vi "LCR Meter Acquire Single_1.vi"() -> ()   [LabVIEW 2021, in "LCR Meter.lvlib"]
doc: "This example shows how to configure a measurement and take a reading."
uses:
  <vilib>/LCR Meter.lvlib
panel:
  out "Boolean":bool
  out "Monitor2 Value":dbl
  out "Monitor1 Value":dbl
  out "Secondary Value":dbl
  out "Primary Value":dbl
  in  "DC Bias Voltage (0)":dbl min=-2.5 max=2.5 step=0.01
  in  "DC Bias":bool caption="BIAS"
  in  "Current Level (1)":dbl=1.0 min=0.1 max=20.0 step=0.01
  in  "Voltage Level (1)":dbl=1.0 min=0.01 max=2.0 step=0.01
  in  "Level Mode":u16(ring) items=["Voltage", "Current"]
  in  "ALC (F: Disable)":bool
  in  "Frequery (1000)":dbl=1000.0 min=10.0 max=300000.0 step=0.01
  in  "Monitor2":i32(ring) items=["OFF", "Z", "D", "Q", "THR", "THD", "R", "X", "G", "B", "Y", "ABS", "PER", "VAC", "IAC"]
  in  "Monitor1":i32(ring) items=["OFF", "Z", "D", "Q", "THR", "THD", "R", "X", "G", "B", "Y", "ABS", "PER", "VAC", "IAC"]
  in  "Speed (0: SLOW)":i32(ring) items=["SLOW", "MED", "FAST"]
  in  "Average (0)":i32 min=0 max=256 step=1
  in  "Auto Range (1: ON)":i32(ring)=1 items=["OFF", "ON", "NOM"]
  in  "Range (0: 0)":i32(ring) items=["0", "1", "2", "3", "4", "5", "6", "7", "8", "MIN", "MAX"]
  in  "Auto LCZ (T: Enable)":bool=TRUE
  in  "Function (0: Cs-Rs)":i32(ring) items=["Cs-Rs", "Cs-D", "Cp-Rp", "Cp-D", "Lp-Rp", "Lp-Q", "Ls-Rs", "Ls-Q", "Rs-Q", "Rp-Q", "R-X", "DCR", "Z-thr", "Z-thd", "Z-D", "Z-Q"]
  in  "Serial Settings:Baud Rate":u32(ring)=115200 items=["9600"=9600, "38400"=38400, "57600"=57600, "115200"=115200]
  in  "VISA resource name":refnum<visa-resource-name>
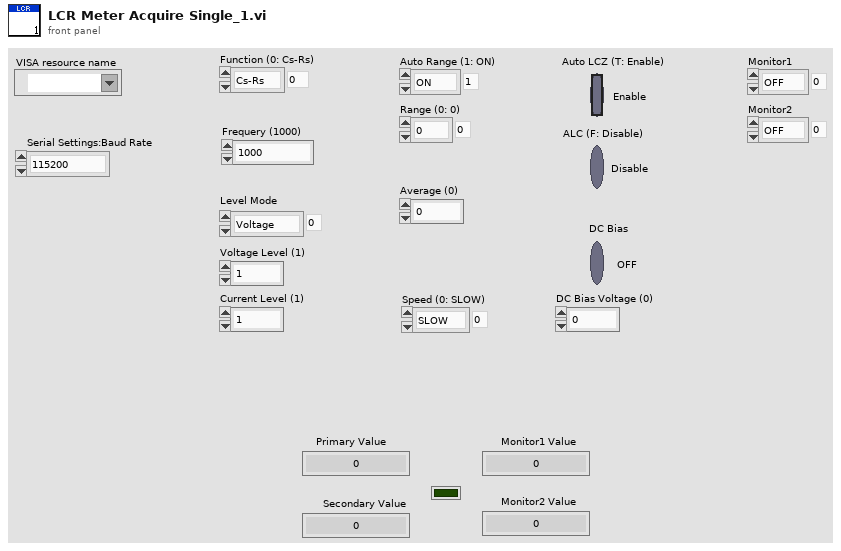
[diagram p1: front panel]
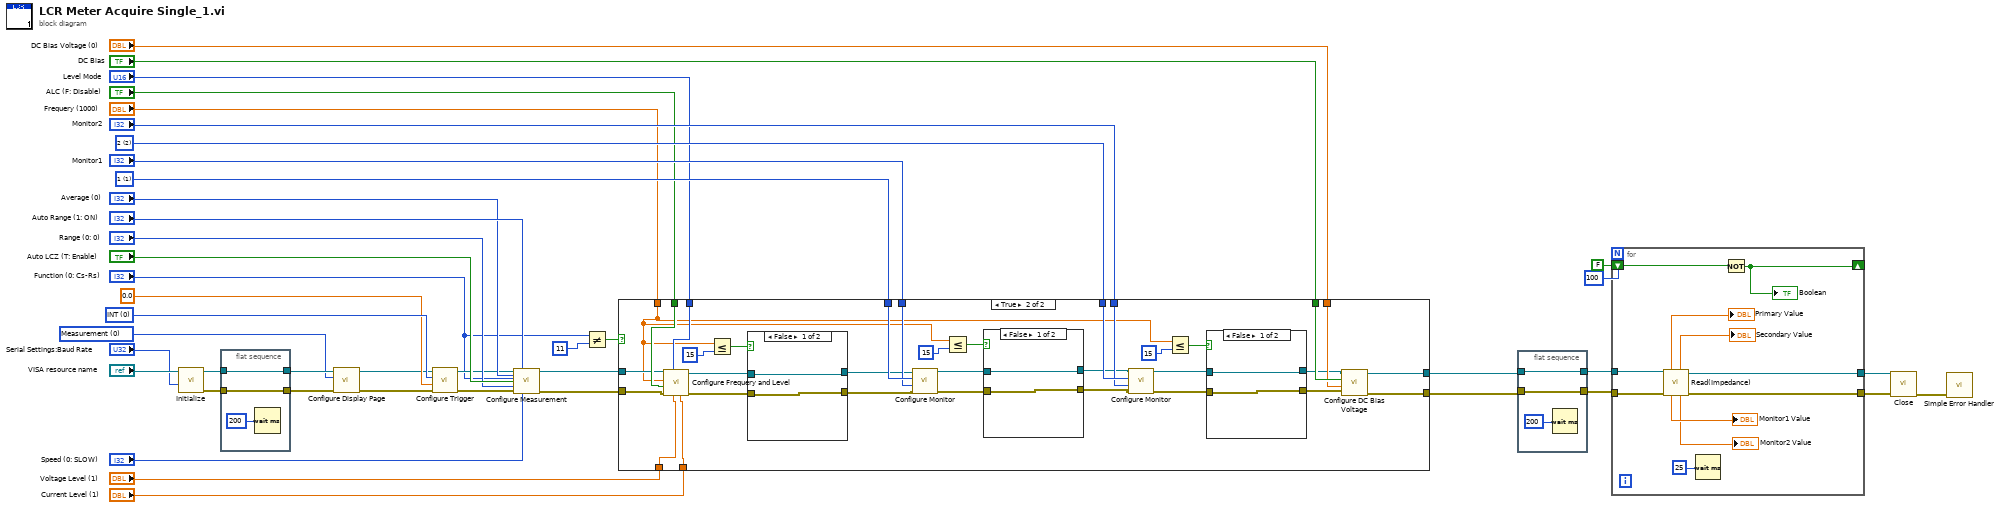
[diagram p0: block diagram]
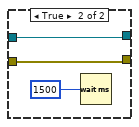
[diagram p3: hidden frame]
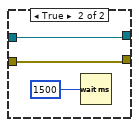
[diagram p4: hidden frame]
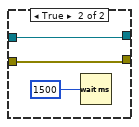
[diagram p5: hidden frame]
diagram:
  w10 = u16 0 items=["Measurement", "Measurement Setup", "BIN Measurement", "BIN Count", "BIN Setup", "LIST Measurement", "LIST Setup", "CORRECTION", "CATALOG", "ENLARGE", "System Config", "System Information"] ("Display Page")
  w22 = 0 items=["INT", "MAN", "EXT", "BUS"] ("Trigger Source (0: INT)")
  w32 = 2 items=["1"=1, "2"=2] ("Monitor (1)")
  w34 = 1 items=["1"=1, "2"=2] ("Monitor (1)")
  n1 = call <vilib>:"Initialize.vi"("Serial Settings:Baud Rate"="Serial Settings:Baud Rate", "VISA resource name"="VISA resource name") -> ("error out"=w13:errorcluster, "VISA resource name out"=w16:refnum<visa-resource-name>)  [unwired: 7 in, 1 out]
  n2 = flat-sequence {
    tunnel: [w46] -> w15
    tunnel: w16 -> [w46]
    tunnel: w13 -> [w45]
    tunnel: [w45] -> w12
    frame #0 {
      n3 = Wait (ms)(milliseconds to wait=u32 200) -> ()  [unwired: 1 out]
    }
  }
  n4 = call <vilib>:"Configure Display Page.vi"("error in"=w12, "Display Page"=w10, "VISA resource name"=w15) -> ("error out"=w11:errorcluster, "VISA resource name out"=w14:refnum<visa-resource-name>)  [unwired: 7 in]
  n5 = call <vilib>:"Configure Trigger.vi"("error in (no error)"=w11, "Trigger Delay (0)"=0.0, "Trigger Source (0: INT)"=w22, "VISA resource name"=w14) -> ("error out"=w23:errorcluster, "VISA resource name out"=w24:refnum<visa-resource-name>)  [unwired: 6 in]
  n6 = call <vilib>:"Configure Measurement.vi"("VISA resource name"=w24, "Auto Range (1: ON)"="Auto Range (1: ON)", "Average (0)"="Average (0)", "Function (0: Cs-Rs)"="Function (0: Cs-Rs)", "Auto LCZ (T: Enable)"="Auto LCZ (T: Enable)", "Range (0: 0)"="Range (0: 0)", "error in (no error)"=w23, "Speed (0: SLOW)"="Speed (0: SLOW)") -> ("VISA resource name out"=w36:refnum<visa-resource-name>, "error out"=w35:errorcluster)  [unwired: 6 in]
  n7 = Not Equal?(x="Function (0: Cs-Rs)", y=11) -> (x != y?=w9:bool)
  n8 = case shown="True" w9 {
    tunnel: w36 -> [w48 w69]
    tunnel: w35 -> [w47 w68]
    tunnel: w34 -> [_ w81]
    tunnel: "Monitor1" -> [_ w80]
    tunnel: w32 -> [_ w79]
    tunnel: "Monitor2" -> [_ w78]
    tunnel: "Frequery (1000)" -> [_ w49]
    tunnel: "ALC (F: Disable)" -> [_ w73]
    tunnel: "Level Mode" -> [_ w72]
    tunnel: "Voltage Level (1)" -> [_ w71]
    tunnel: "Current Level (1)" -> [_ w70]
    tunnel: "DC Bias" -> [_ w77]
    tunnel: "DC Bias Voltage (0)" -> [_ w76]
    tunnel: [w48 w75] -> w5
    tunnel: [w47 w74] -> w4
    frame False {
    }
    frame True {
      n9 = call <vilib>:"Configure Frequery and Level.vi"("Current Level (1)"=w70, "Voltage Level (1)"=w71, "Level Mode"=w72, "error in (no error)"=w68, "ALC (F: Disable)"=w73, "Frequery (1000)"=w49, "VISA resource name"=w69) -> ("error out"=w65:errorcluster, "VISA resource name out"=w64:refnum<visa-resource-name>)  [unwired: 3 in]
      n10 = Less Or Equal?(x=w49, y=15) -> (x <= y?=w66:bool)
      n11 = case shown="False" w66 {
        tunnel: w64 -> [w93 w95]
        tunnel: w65 -> [w92 w94]
        tunnel: [w93 w95] -> w62
        tunnel: [w92 w94] -> w63
        frame False {
        }
        frame True {
          n12 = Wait (ms)(milliseconds to wait=u32 1500) -> ()  [unwired: 1 out]
        }
      }
      n13 = call <vilib>:"Configure Monitor.vi"("error in (no error)"=w63, "Parameter (0: OFF)"=w80, "Monitor (1)"=w81, "VISA resource name"=w62) -> ("error out"=w54:errorcluster, "VISA resource name out"=w57:refnum<visa-resource-name>)  [unwired: 6 in]
      n14 = Less Or Equal?(x=w49, y=15) -> (x <= y?=w60:bool)
      n15 = case shown="False" w60 {
        tunnel: w57 -> [w88 w90]
        tunnel: w54 -> [w87 w89]
        tunnel: [w88 w90] -> w56
        tunnel: [w87 w89] -> w53
        frame False {
        }
        frame True {
          n16 = Wait (ms)(milliseconds to wait=u32 1500) -> ()  [unwired: 1 out]
        }
      }
      n17 = call <vilib>:"Configure Monitor.vi"("error in (no error)"=w53, "Parameter (0: OFF)"=w78, "Monitor (1)"=w79, "VISA resource name"=w56) -> ("error out"=w52:errorcluster, "VISA resource name out"=w55:refnum<visa-resource-name>)  [unwired: 6 in]
      n18 = Less Or Equal?(x=w49, y=15) -> (x <= y?=w58:bool)
      n19 = case shown="False" w58 {
        tunnel: w55 -> [w83 w85]
        tunnel: w52 -> [w82 w84]
        tunnel: [w83 w85] -> w51
        tunnel: [w82 w84] -> w50
        frame False {
        }
        frame True {
          n20 = Wait (ms)(milliseconds to wait=u32 1500) -> ()  [unwired: 1 out]
        }
      }
      n21 = call <vilib>:"Configure DC Bias Voltage.vi"("VISA resource name"=w51, "DC Bias"=w77, "DC Bias Voltage (0)"=w76, "error in (no error)"=w50) -> ("VISA resource name out"=w75:refnum<visa-resource-name>, "error out"=w74:errorcluster)  [unwired: 5 in]
    }
  }
  n22 = flat-sequence {
    tunnel: [w99] -> w3
    tunnel: w5 -> [w99]
    tunnel: w4 -> [w98]
    tunnel: [w98] -> w2
    frame #0 {
      n23 = Wait (ms)(milliseconds to wait=u32 200) -> ()  [unwired: 1 out]
    }
  }
  n24 = for {
    N: 100 -> [_]
    tunnel: w2 -> [w110]
    tunnel: [w104] -> w20
    tunnel: [w103] -> w19
    shift-right: [w101] -> _
    shift-left: FALSE -> [w102]
    tunnel: w3 -> [w100]
    n25 = call <vilib>:"Read(Impedance).vi"("error in (no error)"=w110, "VISA resource name"=w100) -> ("error out"=w103:errorcluster, "VISA resource name out"=w104:refnum<visa-resource-name>, "Monitor2 Value"=→"Monitor2 Value":dbl, "Secondary Value"=→"Secondary Value":dbl, "Monitor1 Value"=→"Monitor1 Value":dbl, "Primary Value"=→"Primary Value":dbl)  [unwired: 3 in, 1 out]
    n26 = Wait (ms)(milliseconds to wait=u32 25) -> ()  [unwired: 1 out]
    n27 = Not(x=w102) -> (.not. x?=w101:bool)
    "Boolean" <- w101
  }
  n28 = call <vilib>:"Close.vi"("error in (no error)"=w19, "VISA resource name"=w20) -> ("error out"=w18:errorcluster)  [unwired: 9 in]
  n29 = call <vilib>:"Simple Error Handler.vi"("error in (no error)"=w18) -> ()  [unwired: 4 in, 5 out]
